vi "Keithley6485.vi"(0 "Measure":refnum<vi>, 2 "Error":refnum<vi>, 3 "Current (A)":refnum<vi>, 4 "Scan in Progress":refnum<vi>, 5 "Samples/Measurement":refnum<vi>, 9 "QUIT":refnum<vi>, 11 "Comm Port":refnum<visa-resource-name>="COM3") -> ()   [LabVIEW 2010]
uses:
  <vilib>/Utility/error.llb/DialogType.ctl
panel:
  in  "Keithley6485":T1(tab)
  out "Status":string
  out "Current":dbl caption="A"
  out "Online":bool
  in  "Enable\nKeithley6485":bool
  in  "Perform Background Correction\nBefore Every Measurement":bool
  in  "Timeout Extension Offset (ms)":u32=1000
  in  "Timeout Extension Rate (ms/sample)":i32=500
  out "Error Message":string=" INSTRUCTIONS:\r\rNormal Use:  When using subVIs that incorporate the error in/error out (or error I/O) structure, place this handler where you want to inform the user of an error, typically at the end of the I/O data path, as the last action of the program.  If the error in error? is ERROR, the handler creates a message describing the error and its source.  If the type of dialog = 1 (default), the message is displayed to the user, who can only acknowedge it.  If the type = 2, the user can acknowledge the message or abort execution; aborting a program with active I/O is not recommended.  If the type = 0, no message is displayed; this is used to process the error programmatically, and the error out cluster elements are wired to individual terminals for that reason.  \r\rOther Use:\n\r\nlocal testing.  To test the error code of a subVI or function that does not have the error I/O structure, you can wire its error code and a source string to the local error code and error source inputs.  If error in error? indicates no error and error code is not equal to 0, the local code and source are substituted for the error in values, and error? is set TRUE (ERROR)."
  # "We have to set an absolute timeout in ms when reading measurements over a serial line.  This needs to be longer for more samples per measurement.  To avoid setting this to the max possible (which is VERY long), the minimum necessary timeout is calculated for every measurement taken.  A linear model is used, where every sample takes \"Rate\" ms to capture and there is \"Offset\" overhead for each measurement.  The 'correct' values for this model are unkown.  If you are getting timeouts, try increasing either one."
  # "Extra Notes ->"
  # "Error out reports Serial I/O errors.\n\nKeithley Error reports error messages returned by the Keithley 6485 picoAmmeter.  Currently, only overvoltage and invalid data errors are supported by this VI."
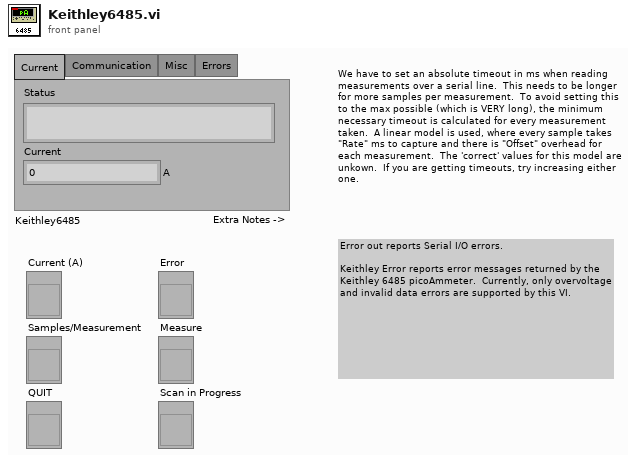
[diagram p1: front panel]
types:
  T1 = enum32{"Current", "Communication", "Misc", "Errors"}
  T2 = typedef "DialogType.ctl" = u16
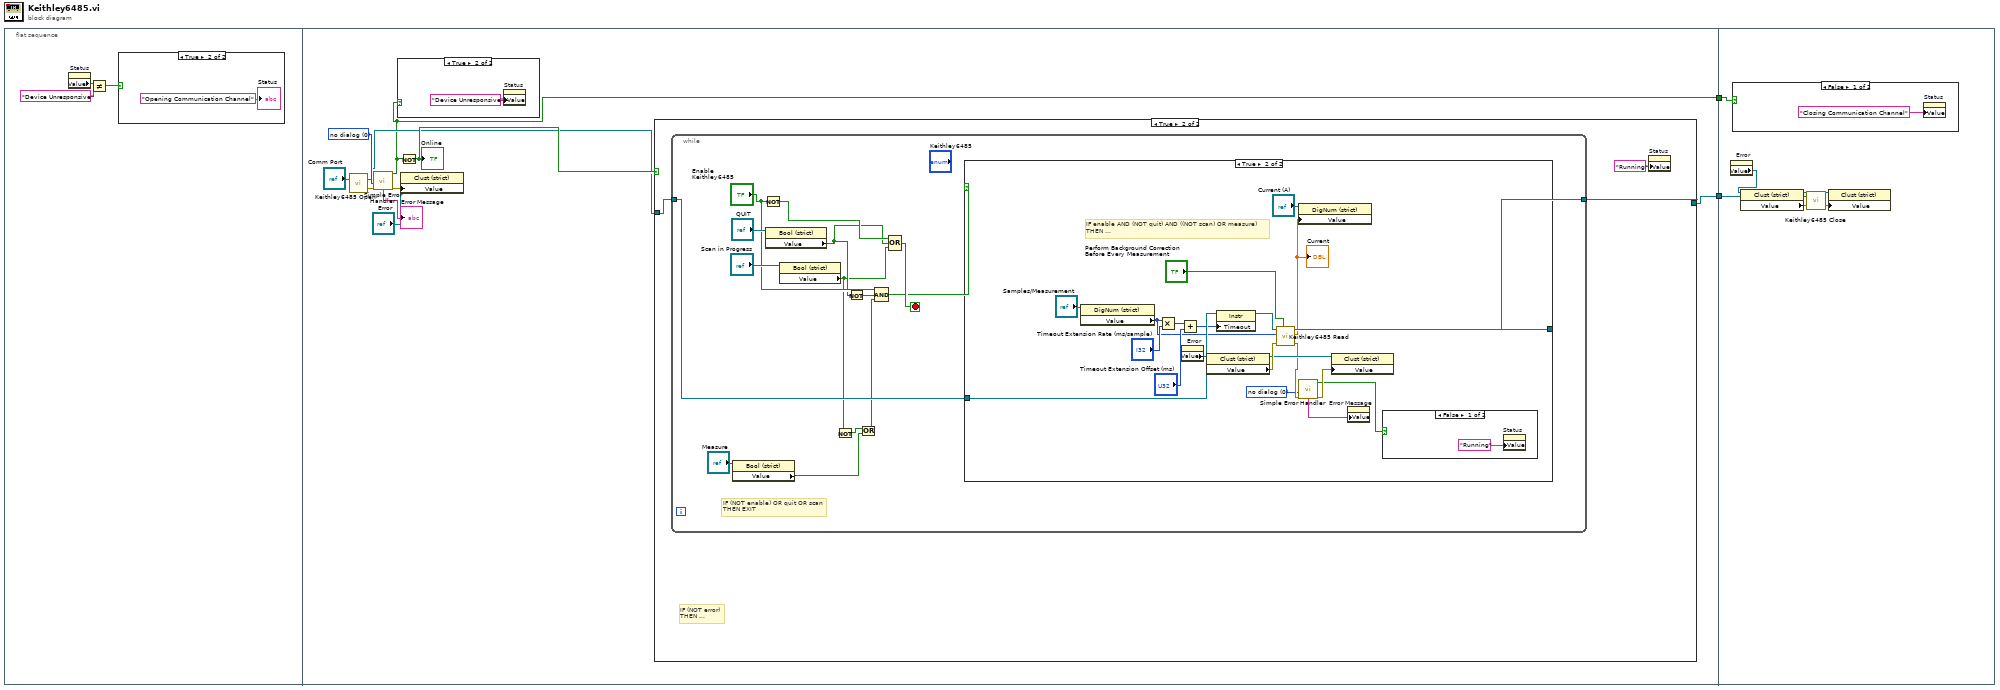
[diagram p0: block diagram]
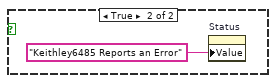
[diagram p6: hidden frame]
diagram:
  n1 = flat-sequence {
    tunnel: [w8] -> w2
    tunnel: [w7] -> w1
    tunnel: w2 -> [w65]
    tunnel: w1 -> [w62]
    frame #0 {
      n2 = property on="Status" class="Str"() -> ("Value"=w5:string)  [unwired: 2 in, 2 out]
      n3 = Not Equal?(x=w5, y="Device Unresponsive" ("Value")) -> (x != y?=w3:bool)
      n4 = case shown="True" w3 {
        frame False {
        }
        frame True {
          "Status" <- "Opening Communication Channel" ("Value")
        }
      }
    }
    frame #1 {
      w13 = T2 0 items=["no dialog", "OK message", "continue or stop message", "OK message + warnings", "continue/stop + warnings"] ("type of dialog (OK msg:1)")
      n5 = call "Keithley6485 Open.vi"("VISA resource name"="Comm Port") -> ("Error out"=w9:errorcluster, "VISA out"=w10:refnum<visa-resource-name>)  [unwired: 1 in]
      n6 = call <vilib>:"Simple Error Handler.vi"("type of dialog (OK msg:1)"=w13, "error in (no error)"=w9) -> ("error?"=w8:bool, "error out"=w11:errorcluster, "message"=→"Error Message":string)  [unwired: 3 in, 2 out]
      n7 = case shown="True" w8 {
        frame False {
        }
        frame True {
          n8 = property on="Status" class="Str"("Value"="Device Unresponsive") -> ()  [unwired: 2 in, 2 out]
        }
      }
      n9 = Not(x=w8) -> (.not. x?=w15:bool)
      "Online" <- w15
      n10 = property on="Property Node" class="Clust (strict)"(reference="Error", "Value"=w11) -> ()  [unwired: 1 in, 2 out]
      n11 = case shown="True" w15 {
        tunnel: w10 -> [w18 w20]
        tunnel: [w18 w21] -> w7
        frame False {
        }
        frame True {
          # "IF (NOT error)\nTHEN ..."
          n12 = while {
            tunnel: w20 -> [w36]
            tunnel: [w35] -> w21
            stop <- w32 stop-if-true
            # "IF (NOT enable) OR quit OR scan\nTHEN EXIT"
            n13 = property on="Property Node" class="Bool (strict)"(reference="Measure") -> ("Value"=w24:bool)  [unwired: 1 in, 2 out]
            n14 = Not(x="Enable\nKeithley6485") -> (.not. x?=w31:bool)
            n15 = property on="Property Node" class="Bool (strict)"(reference="QUIT") -> ("Value"=w28:bool)  [unwired: 1 in, 2 out]
            n16 = property on="Property Node" class="Bool (strict)"(reference="Scan in Progress") -> ("Value"=w27:bool)  [unwired: 1 in, 2 out]
            n17 = Not(x=w27) -> (.not. x?=w26:bool)
            n18 = Not(x=w28) -> (.not. x?=w29:bool)
            n19 = Or(x=w26, y=w24) -> (x .or. y?=w23:bool)
            n20 = Compound Arithmetic op=AND("Enable\nKeithley6485", w29, w23) -> (w22:bool)
            n21 = Compound Arithmetic op=OR(w31, w28, w27) -> (w32:bool)
            n22 = case shown="True" w22 {
              tunnel: w36 -> [w37 w57]
              tunnel: [w37 w56] -> w35
              frame False {
              }
              frame True {
                w40 = T2 0 items=["no dialog", "OK message", "continue or stop message", "OK message + warnings", "continue/stop + warnings"] ("type of dialog (OK msg:1)")
                # "IF enable AND (NOT quit) AND ((NOT scan) OR measure) \nTHEN ..."
                n23 = property on="Property Node" class="DigNum (strict)"(reference="Samples/Measurement") -> ("Value"=w45:i32)  [unwired: 1 in, 2 out]
                n24 = Multiply(x=w45, y="Timeout Extension Rate (ms/sample)") -> (x*y=w54:i32)
                n25 = Add(x=w54, y="Timeout Extension Offset (ms)") -> (x+y=w52:u32)
                n26 = property on="Error" class="LVObjRef (strict)"() -> ("Value"=w44:refnum<vi>)  [unwired: 2 in, 2 out]
                n27 = property on="Property Node" class="Clust (strict)"(reference=w44) -> (reference out=w47:refnum<vi>, "Value"=w50:errorcluster)  [unwired: 1 in, 1 out]
                n28 = property class="Instr"(reference=w57, "Timeout"=w52) -> (reference out=w55:refnum<visa-resource-name>)  [unwired: 1 in, 1 out]
                n29 = call "Keithley6485 Read.vi"("Enable Zero Correction"="Perform Background Correction\nBefore Every Measurement", "error in"=w50, "Sample per measurement"=w45, "VISA in"=w55) -> ("error out"=w42:errorcluster, "Current (A)"=w49:dbl, "VISA out"=w56:refnum<visa-resource-name>)  [unwired: 5 in]
                "Current" <- w49
                n30 = property on="Property Node" class="DigNum (strict)"(reference="Current (A)", "Value"=w49) -> ()  [unwired: 1 in, 2 out]
                n31 = call <vilib>:"Simple Error Handler.vi"("type of dialog (OK msg:1)"=w40, "error in (no error)"=w42) -> ("error?"=w38:bool, "error out"=w41:errorcluster, "message"=w39:string)  [unwired: 3 in, 2 out]
                n32 = property on="Property Node" class="Clust (strict)"(reference=w47, "Value"=w41) -> ()  [unwired: 1 in, 2 out]
                n33 = property on="Error Message" class="Str"("Value"=w39) -> ()  [unwired: 2 in, 2 out]
                n34 = case shown="False" w38 {
                  frame False {
                    n35 = property on="Status" class="Str"("Value"="Running" ("Status")) -> ()  [unwired: 2 in, 2 out]
                  }
                  frame True {
                    n36 = property on="Status" class="Str"("Value"="Keithley6485 Reports an Error" ("Status")) -> ()  [unwired: 2 in, 2 out]
                  }
                }
              }
            }
          }
          n37 = property on="Status" class="Str"("Value"="Running") -> ()  [unwired: 2 in, 2 out]
        }
      }
    }
    frame #2 {
      n38 = property on="Error" class="LVObjRef (strict)"() -> ("Value"=w61:refnum<vi>)  [unwired: 2 in, 2 out]
      n39 = case shown="False" w65 {
        frame False {
          n40 = property on="Status" class="Str"("Value"="Closing Communication Channel") -> ()  [unwired: 2 in, 2 out]
        }
        frame True {
        }
      }
      n41 = property on="Property Node" class="Clust (strict)"(reference=w61) -> (reference out=w60:refnum<vi>, "Value"=w63:errorcluster)  [unwired: 1 in, 1 out]
      n42 = call "Keithley6485 Close.vi"("error in"=w63, "VISA in"=w62) -> ("error out"=w64:errorcluster)  [unwired: 1 in]
      n43 = property on="Property Node" class="Clust (strict)"(reference=w60, "Value"=w64) -> ()  [unwired: 1 in, 2 out]
    }
  }
